vi "svfa_Process Coherent Output Power.vi"(0 "input signal X":waveform(dbl)={"t0"=timestamp(0 s since 1904-01-01), "dt"=1.953125e-05, "Y"=[]}, 1 "input signal Y":waveform(dbl)={"t0"=timestamp(0 s since 1904-01-01), "dt"=1.953125e-05, "Y"=[]}, 2 "window (includes Force_Exp)":T9(ring), 3 "force/exp settings":T8={"force window [%]"=50.0, "exponential window [%]"=10.0} {"exponential window [%]" min=0.0 max=100.0 format="%.2f"; "force window [%]" min=0.0 max=100.0 format="%.2f"}, 4 "averaging parameters":T10={"averaging mode"=enum."No averaging", "weighting mode"=enum."Linear", "number of averages"=10, "linear mode"=enum."Auto restart"}, 5 "error in (no error)":errorcluster, 7 "processing control in":T1(ring)) -> (12 "averages completed":dbl format="%.2f", 13 "processing control out":T1(ring), 14 "coherent output power":cluster{"df":dbl, "df":dbl, dbl[]} {"?" format="%.2f"; "df" format="%.2f"; "df" format="%.2f"}, 15 "coherence":cluster{"df":dbl, "df":dbl, "Coherence":dbl[]} {"Coherence" format="%.2f"; "df" format="%.2f"; "df" format="%.2f"}, 17 "averaging done":bool, 18 "spectrum info":T2={"channel name"="", "description"="", "x-axis units"=0, "spectral info"={"spectrum type"=enum."Power [Magnitude^2]", "linear/dB"=enum."linear", "window"=0, "window size"=0, "FFT size"=0}, "engineering units"=0, "custom label"="", "dB reference [EU]"=0.0, "peak units"=enum."rms", "weighting filter"=0, "spectral density?"=FALSE, "unit label"="", "spectrum skewed?"=FALSE, "complimentary spectrum units"=enum."none"} {"x-axis units" items=["Time (s)"=0, "Frequency-CB (Hz)"=1, "Frequency-CPB (Hz)"=1248, "Frequency-Arbitrary (Hz)"=2357, "Quefrency (s)"=2, "Revolutions (rev)"=3, "Order"=4, "Speed (RPM)"=11, "Speed (rad/s)"=21, "Index"=65535]; "weighting filter" items=["Linear", "A-weighting", "B-weighting", "C-weighting", "ITU-R 468-4", "Dolby", "CCITT", "C-message", "Wb", "Wc", "Wd", "We", "Wf", "Wh", "Wj", "Wk", "Wm", "AES17 20 kHz lowpass", "AES17 40 kHz lowpass", "AES17 20 kHz highpass", "AES17 40 kHz highpass"]; "dB reference [EU]" format="%.2f"; "engineering units" items=["custom..."=0, "V"=1, "A"=21, "C"=30, "pC"=31, "s"=32, "-"=29, "Pa"=2, "N"=20, "g"=3, "m/s^2"=4, "m/s"=5, "m"=6, "mm/s"=12, "mm"=13, "micron/s"=14, "micron"=15, "in/s^2"=7, "in/s"=8, "in"=9, "mil/s"=10, "mil"=11, "rad/s^2"=16, "rad/s"=17, "rad"=18, "deg/s^2"=26, "deg/s"=27, "deg"=28, "RPM"=22, "cycle/s^2"=23, "Hz"=24, "cycle"=25, "strain"=19]; "spectral info"."window" items=["None "=0, "Hanning"=1, "Hamming"=2, "Blackman-Harris"=3, "Exact Blackman"=4, "Blackman"=5, "Flat Top"=6, "4 Term B-Harris "=7, "7 Term B-Harris"=8, "Low Sidelobe"=9, "Force - Exponential"=10, "Gaussian"=62]}, 19 "error out":errorcluster)   [LabVIEW 2017]
uses:
  <vilib>/addons/_NISVFA/_Shared subVIs/Controls/svc_Spectrum Info.ctl
  <vilib>/addons/_NISVFA/_Shared subVIs/Controls/svc_X-Axis Units.ctl
  <vilib>/addons/_NISVFA/_Shared subVIs/Controls/svc_Spectrum Type.ctl
  <vilib>/addons/_NISVFA/_Shared subVIs/Controls/svc_Engineering Units Text Ring.ctl
  <vilib>/addons/_NISVFA/_Shared subVIs/Controls/svc_Weighting Filter Text Ring.ctl
  <vilib>/addons/_NISVFA/_Shared subVIs/Controls/svc_Complimentary Spectrum Units.ctl
  <vilib>/addons/_NISVFA/_Shared subVIs/Windowing/svfa_Scaled Time Domain Window (1 Ch).vi
  <vilib>/addons/_NISVFA/_Shared subVIs/Windowing/svfa_Scaled Time Domain Window (Array).vi
  <vilib>/Analysis/4window.llb/Force Window.vi
  <vilib>/Analysis/4window.llb/Force Window (DBL).vi
  <vilib>/Analysis/4window.llb/Exponential Window.vi
  <vilib>/Analysis/4window.llb/Exponential Window (DBL).vi
  <vilib>/Utility/error.llb/Error Cluster From Error Code.vi
  <vilib>/Analysis/0measdsp.llb/Scaled Time Domain Window.vi
  <vilib>/Analysis/0measdsp.llb/Scaled Time Domain Window (DBL).vi
  <vilib>/addons/_NISVFA/_Spectrum Processing/subVIs/svfa_Spectrum Info Window to windowTd Type Def.vi
  <vilib>/addons/_NISVFA/_Shared subVIs/Common/svc_Window Parameters.vi
  <vilib>/addons/_NISVFA/_Shared subVIs/Common/svc_Get Window Info.vi
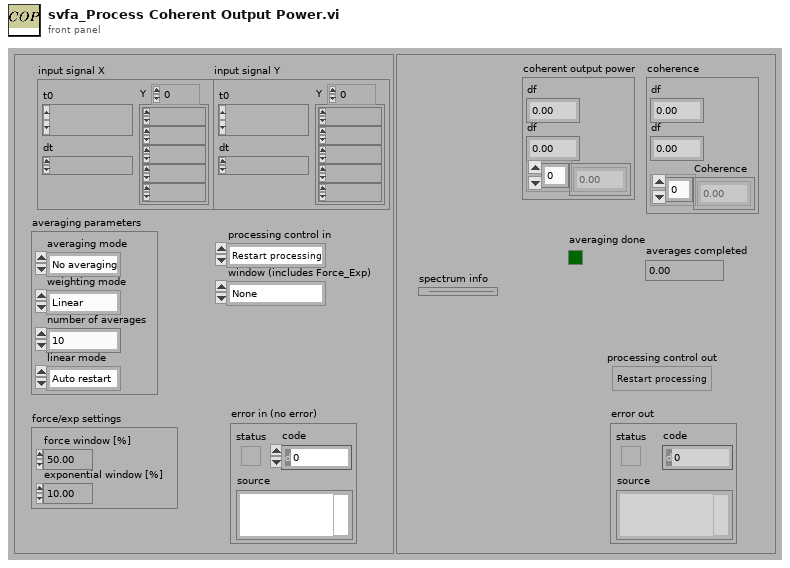
[diagram p1: front panel]
types:
  T1 = enum16{"Restart processing", "Continue processing", "Skip processing"}
  T2 = typedef "svc_Spectrum Info.ctl" = cluster{"channel name":string, "description":string, "x-axis units":T3, "spectral info":cluster{"spectrum type":T4, "linear/dB":enum16{"linear", "dB"}, "window":u16, "window size":i32, "FFT size":i32}, "engineering units":T5, "custom label":string, "dB reference [EU]":dbl, "peak units":enum16{"rms", "peak", "peak-peak"}, "weighting filter":T6, "spectral density?":bool, "unit label":string, "spectrum skewed?":bool, "complimentary spectrum units":T7}
  T3 = typedef "svc_X-Axis Units.ctl" = u16
  T4 = typedef "svc_Spectrum Type.ctl" = enum16{"FFT Spectrum [complex]", "Amplitude [Magnitude]", "Power [Magnitude^2]", "Cross Spectrum [complex]", "Frequency Response [Complex]"}
  T5 = typedef "svc_Engineering Units Text Ring.ctl" = u16
  T6 = typedef "svc_Weighting Filter Text Ring.ctl" = u16
  T7 = typedef "svc_Complimentary Spectrum Units.ctl" = enum16{"none", "radians", "degrees", "cycles", "imaginary"}
  T8 = cluster{"force window [%]":dbl, "exponential window [%]":dbl}
  T9 = enum16{"None ", "Hanning", "Hamming", "Blackman-Harris", "Exact Blackman", "Blackman", "Flat Top", "4 Term B-Harris ", "7 Term B-Harris", "Low Sidelobe", "Force - Exponential"}
  T10 = cluster{"averaging mode":enum16{"No averaging", "Vector averaging", "RMS averaging", "Peak hold"}, "weighting mode":enum16{"Linear", "Exponential"}, "number of averages":u32, "linear mode":enum16{"One shot", "Auto restart"}}
  T11 = typedef "svc_Window [Dual FFT].ctl" = u32
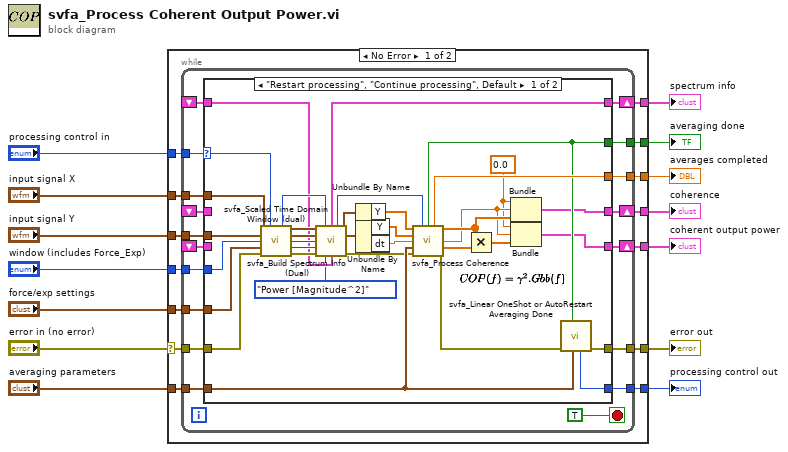
[diagram p0: block diagram]
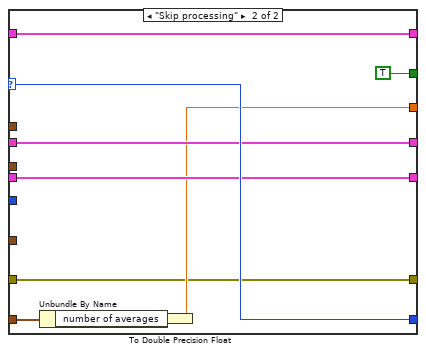
[diagram p2: hidden frame]
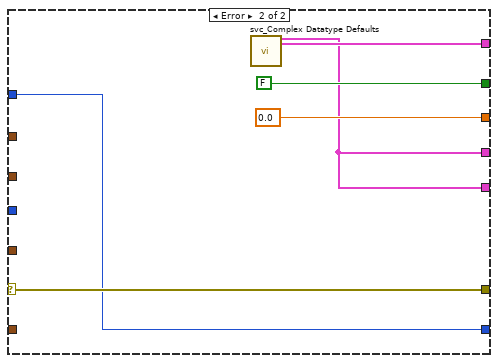
[diagram p3: hidden frame]
diagram:
  n1 = case shown="No Error" "error in (no error)" {
    selector: "error in (no error)" -> [w26 w96]
    tunnel: "input signal X" -> [w22 _]
    tunnel: "input signal Y" -> [w27 _]
    tunnel: "averaging parameters" -> [w25 _]
    tunnel: [w15 w91] -> w9
    tunnel: [w24 FALSE ("averaging done")] -> w8
    tunnel: [w28 0.0 ("averages completed")] -> w7
    tunnel: "processing control in" -> [w21 w93]
    tunnel: [w23 w93] -> w5
    tunnel: [w16 w91] -> w4
    tunnel: [w17 w92] -> w3
    tunnel: "window (includes Force_Exp)" -> [w20 _]
    tunnel: "force/exp settings" -> [w19 _]
    tunnel: [w18 w96] -> w13
    frame No Error {
      n2 = while {
        shift-left: _ -> [w29]
        shift-right: [w32] -> w15
        shift-left: _ -> [w30]
        shift-right: [w33] -> w16
        shift-left: _ -> [w31]
        shift-right: [w34] -> w17
        tunnel: [w37] -> w18
        tunnel: w19 -> [w38]
        tunnel: w20 -> [w39]
        tunnel: w21 -> [w35]
        tunnel: w22 -> [w40]
        tunnel: [w41] -> w23
        tunnel: [w42] -> w24
        tunnel: w25 -> [w43]
        tunnel: w26 -> [w44]
        tunnel: w27 -> [w45]
        tunnel: [w46] -> w28
        stop <- TRUE stop-if-true
        n3 = case shown="\"Restart processing\", \"Continue processing\", Default" w35 {
          selector: w35 -> [w61 w89]
          tunnel: [w80 w83] -> w46
          tunnel: w45 -> [w77 _]
          tunnel: w44 -> [w75 w82]
          tunnel: w43 -> [w74 w85]
          tunnel: [w73 TRUE ("averaging done")] -> w42
          tunnel: [w72 w89] -> w41
          tunnel: w40 -> [w71 _]
          tunnel: w39 -> [w49 _]
          tunnel: w38 -> [w70 _]
          tunnel: [w50 w87] -> w32
          tunnel: [w54 w88] -> w33
          tunnel: [w66 w82] -> w37
          tunnel: [w62 w90] -> w34
          tunnel: w31 -> [w48 w90]
          tunnel: w30 -> [_ w88]
          tunnel: w29 -> [_ w87]
          frame "Restart processing", "Continue processing", Default {
            w51 = 0.0 ("df")
            n4 = call <vilib>:"svfa_Scaled Time Domain Window (dual).vi"("Signal in [X]"=w71, "processing control"=w61, "Signal in [Y]"=w77, "window"=w49, "force/exp settings"=w70, "error in (no error)"=w75) -> ("dup processing control"=w64:T1, "Windowed signal [X]"=w79:waveform(dbl), "Windowed signal [Y]"=w78:waveform(dbl), "window"=w69:T11, "window size"=w68:i32, "error out"=w76:errorcluster)  [unwired: 3 in, 1 out]
            n5 = call <vilib>:"svfa_Build Spectrum Info (Dual).vi"("scaled signal  X [EU]"=w79, "processing control"=w64, "scaled signal  Y [EU]"=w78, "window"=w69, "window size"=w68, "error in (no error)"=w76, "spectrum type"=svc_Spectrum_Type."Power [Magnitude^2]", "spectrum info in"=w48) -> ("spectrum info out"=w62:T2, "dup processing control"=w63:T1, "dup scaled signal  X [EU]"=w59:waveform(dbl), "dup scaled signal  Y [EU]"=w60:waveform(dbl), "error out"=w67:errorcluster)  [unwired: 3 in]
            n6 = Unbundle By Name ("Get Waveform Components")(w59) -> ("Y"=w56:dbl[])
            n7 = Unbundle By Name ("Get Waveform Components")(w60) -> ("Y"=w57:dbl[], "dt"=w58:dbl)
            n8 = call <vilib>:"svfa_Process Coherence.vi"("Windowed signal [X]"=w56, "processing control"=w63, "Windowed signal [Y]"=w57, "dt"=w58, "averaging parameters"=w74, "error in (no error)"=w67) -> ("averaging done"=w73:bool, "averages completed"=w80:dbl, "Coherence"=w55:dbl[], "df"=w52:dbl, "<Gyy>"=w81:dbl[], "error out"=w65:errorcluster)  [unwired: 1 in, 3 out]
            n9 = Multiply(x=w55, y=w81) -> (x*y=w53:dbl[])
            n10 = Bundle("df"=w51, "df"=w52, "Coherence"=w55) -> (w54:cluster{"df":dbl, "df":dbl, "Coherence":dbl[]})  [unwired: 1 in]
            n11 = Bundle("df"=w51, "df"=w52, w53) -> (w50:cluster{"df":dbl, "df":dbl, dbl[]})  [unwired: 1 in]
            n12 = call <vilib>:"svfa_Linear OneShot or AutoRestart Averaging Done.vi"("averaging parameters"=w74, "averaging done"=w73, "error in (no error)"=w65) -> ("error out"=w66:errorcluster, "processing control"=w72:T1)  [unwired: 7 in]
          }
          frame "Skip processing" {
            n13 = Unbundle By Name(w85) -> ("number of averages"=w84:u32)
            n14 = To Double Precision Float(number=w84) -> (double precision float=w83:dbl)
          }
        }
      }
    }
    frame Error {
      n15 = call <vilib>:"svc_Complex Datatype Defaults.vi"() -> ("empty spectrum"=w91:cluster{"f0":dbl, "df":dbl, "magnitude":dbl[]}, "dead spectrum info"=w92:T2)  [unwired: 11 in, 7 out]
    }
  }
  "error out" <- w13
  "coherent output power" <- w9
  "averaging done" <- w8
  "averages completed" <- w7
  "spectrum info" <- w3
  "processing control out" <- w5
  "coherence" <- w4
